vi "Find Lines.vi"(6 "Edge Options":T2={"Edge Polarity"=0, "Kernel Size"=13, "Width"=13, "Minimum Edge Strength"=20.0, "Interpolation Type"=enum."Zero Order", "Data Processing Method"=enum."Average"} {"Edge Polarity" items=["All Edges", "Rising Edges", "Falling Edges"]}, 7 "Line Options":T1={"Number of Lines"=1, "Type"=enum."Best Edge Rake", "Min. Score"=0.0, "Max. Score"=1024.0, "Orientation"=0.0, "Angle Range"=90.0, "Angle Tolerance"=1.0, "Step Size"=33, "Min. SNR (db)"=0.0, "Min. Points (%)"=25.0, "Hough Iterations"=5}, 8 "error in":errorcluster, 9 "Search Direction":u32(ring)=2 items=["Left to Right", "Right to Left", "Top to Bottom", "Bottom to Top"], 10 "ROI":T3={"Global Rectangle"=[671, 515, 948, 693], "Contours"=[{"ID"=enum."External", "Type"=12, "Coordinates"=[671, 515, 948, 693, 0]}]} {"Contours"."Type" items=["No Selection", "Point", "Line", "Rectangle", "Oval", "Polygon", "Freehand Region", "Annulus", "Unused2", "Unused3", "Broken Line", "Freehand Line", "Rotated Rectangle"]}, 11 "Image In":T5) -> (0 "error out":errorcluster, 2 "Straight Edges":T4(array[cluster]) {"Point2 (Real-World)"."Y" format="%.2f"; "Point2 (Real-World)"."X" format="%.2f"; "Point1 (Real-World)"."Y" format="%.2f"; "Point1 (Real-World)"."X" format="%.2f"; "Point2 (Pixels)"."Y" format="%.2f"; "Point2 (Pixels)"."X" format="%.2f"; "Point1 (Pixels)"."Y" format="%.2f"; "Point1 (Pixels)"."X" format="%.2f"}, 3 "Image Out":T5)   [LabVIEW 2013]
uses:
  <vilib>/vision/Image Controls.llb/IMAQ Image.ctl
  <vilib>/vision/NI_Vision_Development_Module.lvlib
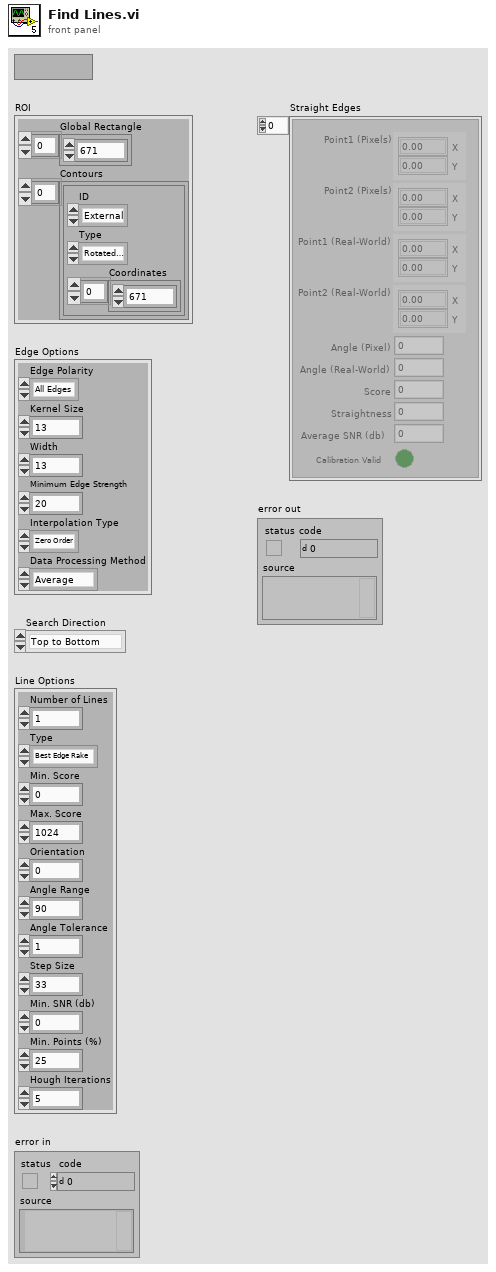
[diagram p1: front panel]
types:
  T1 = cluster{"Number of Lines":i32, "Type":enum32{"First Edge Rake", "Best Edge Rake", "Hough Edge Rake", "First Edge Projection", "Best Edge Projection"}, "Min. Score":dbl, "Max. Score":dbl, "Orientation":dbl, "Angle Range":dbl, "Angle Tolerance":dbl, "Step Size":u32, "Min. SNR (db)":dbl, "Min. Points (%)":dbl, "Hough Iterations":i32}
  T2 = cluster{"Edge Polarity":u32, "Kernel Size":u32, "Width":u32, "Minimum Edge Strength":sgl, "Interpolation Type":enum32{"Zero Order", "Bilinear", "Quadratic", "Cubic", "Bilinear Fixed"}, "Data Processing Method":enum32{"Average", "Median"}}
  T3 = cluster{"Global Rectangle":i32[], "Contours":cluster{"ID":enum32{"External", "Internal"}, "Type":u32, "Coordinates":i32[]}[]}
  T4 = cluster{"Point1 (Pixels)":cluster{"X":sgl, "Y":sgl}, "Point2 (Pixels)":cluster{"X":sgl, "Y":sgl}, "Point1 (Real-World)":cluster{"X":sgl, "Y":sgl}, "Point2 (Real-World)":cluster{"X":sgl, "Y":sgl}, "Angle (Pixel)":dbl, "Angle (Real-World)":dbl, "Score":dbl, "Straightness":dbl, "Average SNR (db)":dbl, "Calibration Valid":bool}[]
  T5 = typedef "IMAQ Image.ctl" = refnum<image>
  T6 = cluster{"Show Search Area":bool, "Show Search Lines":bool, "Show Edges Found":bool, "Show Result":bool}
  T7 = typedef "Search Line.ctl" = cluster{"Start Point":cluster{"X":sgl, "Y":sgl}, "End Point":cluster{"X":sgl, "Y":sgl}, "Edge Info":T8[], "Edge Map":dbl[], "Calibration Valid":bool}
  T8 = typedef "Edge New.ctl" = cluster{"Location (Pixel)":cluster{"X":sgl, "Y":sgl}, "Location (Real-World)":cluster{"X":sgl, "Y":sgl}, "Distance (Pixel)":dbl, "Distance (Real-World)":dbl, "Strength":dbl, "Noise":dbl, "Rising?":bool}
  T9 = cluster{"Straight Edges":cluster{"Point1 (Pixels)":cluster{"X":sgl, "Y":sgl}, "Point2 (Pixels)":cluster{"X":sgl, "Y":sgl}, "Point1 (Real-World)":cluster{"X":sgl, "Y":sgl}, "Point2 (Real-World)":cluster{"X":sgl, "Y":sgl}, "Angle (Pixel)":dbl, "Angle (Real-World)":dbl, "Score":dbl, "Straightness":dbl, "Average SNR (db)":dbl, "Calibration Valid":bool}[], "Search Lines Information":T7[], "Used Edges":cluster{"Edge Information":T8[]}[]}
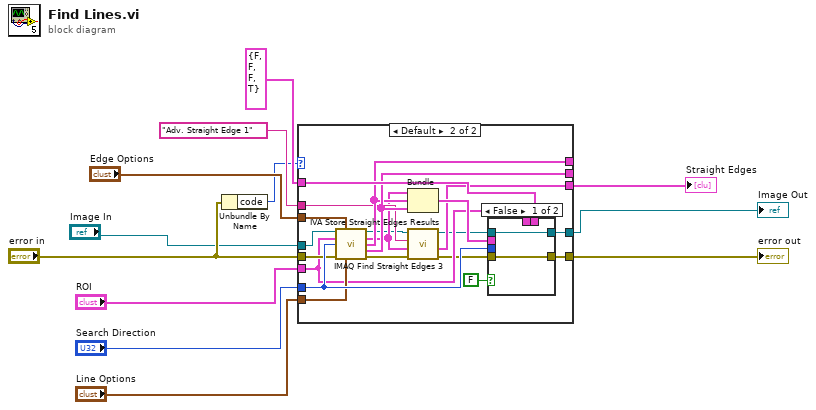
[diagram p0: block diagram]
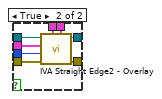
[diagram p3: hidden frame]
diagram:
  n1 = Unbundle By Name("error in") -> ("code"=w5:i32)
  n2 = case shown="Default" w5 {
    tunnel: "Edge Options" -> [_ w33]
    tunnel: "Search Direction" -> [_ w32]
    tunnel: "Line Options" -> [_ w31]
    tunnel: "Image In" -> [w13 w14]
    tunnel: [w13 w29] -> w2
    tunnel: [_ w28] -> w1
    tunnel: T6 {"Show Search Area"=FALSE, "Show Search Lines"=FALSE, "Show Edges Found"=FALSE, "Show Result"=TRUE} ("Setup") -> [_ w27]
    tunnel: "error in" -> [_ w26]
    tunnel: [_ w25] -> _
    tunnel: [_ w24] -> _
    tunnel: "Adv. Straight Edge 1" ("Step Name") -> [_ w23]
    tunnel: [_ w22] -> w7
    tunnel: "ROI" -> [_ w20]
    frame -1074396199, -1074396198 {
      # "Discard Coordinate System Error"
    }
    frame Default {
      n3 = call "IMAQ Find Straight Edges 3"("Image"=w14, "Edge Options"=w33, "ROI Descriptor"=w20, "Search Direction"=w32, "error in (no error)"=w26, "Line Options"=w31) -> ("Image (duplicate)"=w19:T5, "Straight Edges"=w21:T4, "Search Lines Information"=w24:T7[], "Used Edges"=w25:cluster{"Edge Information":T8[]}[], "error out"=w17:errorcluster)  [unwired: 1 in, 4 out]
      n4 = Bundle("Straight Edges"=w21, "Search Lines Information"=w24, "Used Edges"=w25) -> (w30:T9)  [unwired: 1 out]
      n5 = call <vilib>:"IVA Store Straight Edges Results.vi"("error in (no error)"=w17, "Straight Edges"=w21, "Step Name"=w23, "Image in"=w19) -> ("error out"=w16:errorcluster, "Straight Edges dup"=w22:T4, "Image dup"=w18:T5)  [unwired: 5 out]
      n6 = case shown="False" FALSE {
        tunnel: w32 -> [_ w43]
        tunnel: w30 -> [_ w42]
        tunnel: [w35 w41] -> w29
        tunnel: [w34 w40] -> w28
        tunnel: w27 -> [_ w39]
        tunnel: w20 -> [_ w38]
        tunnel: w18 -> [w35 w37]
        tunnel: w16 -> [w34 w36]
        frame False {
        }
        frame True {
          n7 = call <vilib>:"IVA Straight Edge2 - Overlay.vi"("Setup"=w39, "Search Area"=w38, "error in (no error)"=w36, "Scan Direction"=w43, "Edge Results"=w42, "Image In"=w37) -> ("error out"=w40:errorcluster, "Image Out"=w41:T5)  [unwired: 1 in, 3 out]
        }
      }
    }
  }
  "Image Out" <- w2
  "error out" <- w1
  "Straight Edges" <- w7
